vi "DAQmx Timing (Burst Export Clock).vi"(0 "task/channels in":refnum<k21>, 1 "sample mode":i32(ring)=10178 items=["Finite Samples"=10178, "Continuous Samples"=10123, "Hardware Timed Single Point"=12522], 2 "samples per channel":i32=1000, 5 "sample clock rate":dbl=1000.0, 7 "sample clock output terminal":tag, 9 "sample clock pulse polarity":i32(ring)=10095 items=["Active High"=10095, "Active Low"=10096], 11 "error in":errorcluster, 12 "pause when":i32(ring)=10192 items=["High"=10192, "Low"=10214], 13 "ready for transfer event active level":i32(ring)=10095 items=["Active High"=10095, "Active Low"=10096]) -> (4 "task out":refnum<k21>, 15 "error out":errorcluster)   [LabVIEW 2020]
doc: "Configures when the DAQ device transfers data to a peripheral device, using the onboard Sample Clock of the DAQ device to control burst handshake timing and exporting that clock for use by the peripheral device."
uses:
  nilvaiu.dll
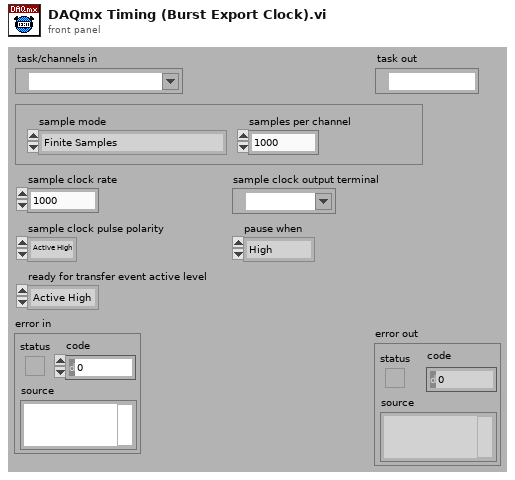
[diagram p1: front panel]
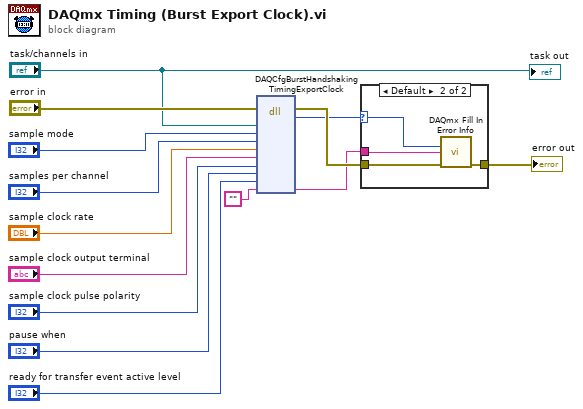
[diagram p0: block diagram]
diagram:
  n1 = dll-call lib="nilvaiu.*" fn="DAQCfgBurstHandshakingTimingExportClock"(error in="error in", "taskID"="task/channels in", "sampleMode"="sample mode", "samplesPerChannel"="samples per channel", "rate"="sample clock rate", "sampleClockOutputTerm"="sample clock output terminal", "sampleClockPulsePolarity"="sample clock pulse polarity", "pauseWhen"="pause when", "readyForTransferEventActiveLevel"="ready for transfer event active level", "extendedErrorInfo"="") -> (error out=w11:errorcluster, "return type"=w10:i32, "extendedErrorInfo"=w2:string)  [unwired: 4 in, 7 out]
  n2 = case shown="Default" w10 {
    selector: w10 -> [_ w17]
    tunnel: w11 -> [w15 w19]
    tunnel: [w15 w18] -> w13
    tunnel: w2 -> [_ w16]
    frame 0 {
    }
    frame Default {
      n3 = call "DAQmx Fill In Error Info.vi"("status code"=w17, "extended error info"=w16, "error in"=w19) -> ("error out"=w18:errorcluster)  [unwired: 1 in, 11 out]
    }
  }
  "error out" <- w13
  "task out" <- "task/channels in"
